vi "CheckArmAngle.vi"(10 "Tolerance  Angle Difference":dbl, 11 "Target Angle":dbl) -> (2 "Positive /Negative":bool, 3 "Outside Tolerance":bool)   [LabVIEW 2013]
doc: "Checks the angle of a motor with a target angle and tolerance angle difference to output a true or false for a positive/ negative movement, and outputs a true or false if it is te range of the outside tolerance."
panel:
  out "Angle Difference":dbl
  # "Positive (true) means raise, negative (false) means lower"
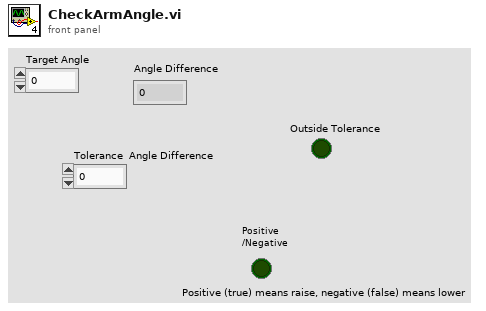
[diagram p1: front panel]
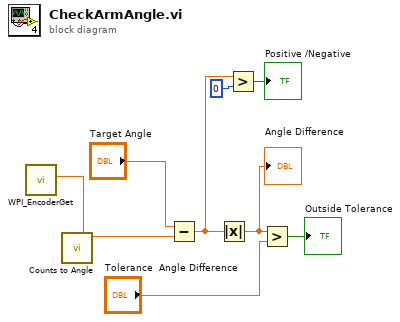
[diagram p0: block diagram]
diagram:
  n1 = call <vilib>:"WPI_EncoderGet.vi"() -> ("Distance"=w2:dbl)  [unwired: 6 in, 5 out]
  n2 = call "Counts to Angle.vi"("Input Counts"=w2) -> ("Output Angle"=w1:dbl)  [unwired: 10 in]
  n3 = Subtract(x="Target Angle", y=w1) -> (x-y=w5:dbl)
  n4 = Absolute Value(x=w5) -> (abs(x)=w8:dbl)
  "Angle Difference" <- w8
  n5 = Greater?(x=w5, y=0) -> (0:→"Positive /Negative":bool)
  n6 = Greater?(x=w8, y="Tolerance  Angle Difference") -> (0:→"Outside Tolerance":bool)
